vi "test TCX read (installed 71).vi"() -> ()   [LabVIEW 2011] (continued)
Position><AltitudeMeters>72.236</AltitudeMeters><DistanceMeters>5473.570</DistanceMeters><Cadence>72</Cadence><Extensions><TPX xmlns=\"http://www.garmin.com/xmlschemas/ActivityExtension/v2\"><Watts>158</Watts></TPX></Extensions></Trackpoint><Trackpoint><Time>2008-03-03T13:58:05Z</Time><Position><LatitudeDegrees>35.874487</LatitudeDegrees><LongitudeDegrees>-78.914089</LongitudeDegrees></Position><AltitudeMeters>72.236</AltitudeMeters><DistanceMeters>5483.258</DistanceMeters><Cadence>72</Cadence><Extensions><TPX xmlns=\"http://www.garmin.com/xmlschemas/ActivityExtension/v2\"><Watts>160</Watts></TPX></Extensions></Trackpoint><Trackpoint><Time>2008-03-03T13:58:06Z</Time><Position><LatitudeDegrees>35.874409</LatitudeDegrees><LongitudeDegrees>-78.914037</LongitudeDegrees></Position><AltitudeMeters>71.755</AltitudeMeters><DistanceMeters>5493.159</DistanceMeters><Cadence>73</Cadence><Extensions><TPX xmlns=\"http://www.garmin.com/xmlschemas/ActivityExtension/v2\"><Watts>157</Watts></TPX></Extensions></Trackpoint><Trackpoint><Time>2008-03-03T13:58:07Z</Time><Position><LatitudeDegrees>35.874330</LatitudeDegrees><LongitudeDegrees>-78.913985</LongitudeDegrees></Position><AltitudeMeters>72.236</AltitudeMeters><DistanceMeters>5503.068</DistanceMeters><Cadence>74</Cadence><Extensions><TPX xmlns=\"http://www.garmin.com/xmlschemas/ActivityExtension/v2\"><Watts>162</Watts></TPX></Extensions></Trackpoint><Trackpoint><Time>2008-03-03T13:58:08Z</Time><Position><LatitudeDegrees>35.874258</LatitudeDegrees><LongitudeDegrees>-78.913934</LongitudeDegrees></Position><AltitudeMeters>71.275</AltitudeMeters><DistanceMeters>5512.351</DistanceMeters><Cadence>75</Cadence><Extensions><TPX xmlns=\"http://www.garmin.com/xmlschemas/ActivityExtension/v2\"><Watts>156</Watts></TPX></Extensions></Trackpoint><Trackpoint><Time>2008-03-03T13:58:09Z</Time><Position><LatitudeDegrees>35.874185</LatitudeDegrees><LongitudeDegrees>-78.913883</LongitudeDegrees></Position><AltitudeMeters>71.755</AltitudeMeters><DistanceMeters>5521.553</DistanceMeters><Cadence>76</Cadence><Extensions><TPX xmlns=\"http://www.garmin.com/xmlschemas/ActivityExtension/v2\"><Watts>154</Watts></TPX></Extensions></Trackpoint><Trackpoint><Time>2008-03-03T13:58:10Z</Time><Position><LatitudeDegrees>35.874110</LatitudeDegrees><LongitudeDegrees>-78.913831</LongitudeDegrees></Position><AltitudeMeters>71.755</AltitudeMeters><DistanceMeters>5531.185</DistanceMeters><Cadence>76</Cadence><Extensions><TPX xmlns=\"http://www.garmin.com/xmlschemas/ActivityExtension/v2\"><Watts>152</Watts></TPX></Extensions></Trackpoint><Trackpoint><Time>2008-03-03T13:58:11Z</Time><Position><LatitudeDegrees>35.874038</LatitudeDegrees><LongitudeDegrees>-78.913777</LongitudeDegrees></Position><AltitudeMeters>71.755</AltitudeMeters><DistanceMeters>5540.583</DistanceMeters><Cadence>76</Cadence><Extensions><TPX xmlns=\"http://www.garmin.com/xmlschemas/ActivityExtension/v2\"><Watts>151</Watts></TPX></Extensions></Trackpoint><Trackpoint><Time>2008-03-03T13:58:12Z</Time><Position><LatitudeDegrees>35.873964</LatitudeDegrees><LongitudeDegrees>-78.913723</LongitudeDegrees></Position><AltitudeMeters>71.755</AltitudeMeters><DistanceMeters>5550.070</DistanceMeters><Cadence>76</Cadence><Extensions><TPX xmlns=\"http://www.garmin.com/xmlschemas/ActivityExtension/v2\"><Watts>149</Watts></TPX></Extensions></Trackpoint><Trackpoint><Time>2008-03-03T13:58:13Z</Time><Position><LatitudeDegrees>35.873889</LatitudeDegrees><LongitudeDegrees>-78.913669</LongitudeDegrees></Position><AltitudeMeters>71.275</AltitudeMeters><DistanceMeters>5559.694</DistanceMeters><Cadence>76</Cadence><Extensions><TPX xmlns=\"http://www.garmin.com/xmlschemas/ActivityExtension/v2\"><Watts>151</Watts></TPX></Extensions></Trackpoint><Trackpoint><Time>2008-03-03T13:58:14Z</Time><Position><LatitudeDegrees>35.873816</LatitudeDegrees><LongitudeDegrees>-78.913616</LongitudeDegrees></Position><AltitudeMeters>71.275</AltitudeMeters><DistanceMeters>5569.145</DistanceMeters><Cadence>75</Cadence><Extensions><TPX xmlns=\"http://www.garmin.com/xmlschemas/ActivityExtension/v2\"><Watts>155</Watts></TPX></Extensions></Trackpoint><Trackpoint><Time>2008-03-03T13:58:15Z</Time><Position><LatitudeDegrees>35.873721</LatitudeDegrees><LongitudeDegrees>-78.913558</LongitudeDegrees></Position><AltitudeMeters>71.275</AltitudeMeters><DistanceMeters>5580.802</DistanceMeters><Cadence>75</Cadence><Extensions><TPX xmlns=\"http://www.garmin.com/xmlschemas/ActivityExtension/v2\"><Watts>155</Watts></TPX></Extensions></Trackpoint><Trackpoint><Time>2008-03-03T13:58:16Z</Time><Position><LatitudeDegrees>35.873636</LatitudeDegrees><LongitudeDegrees>-78.913501</LongitudeDegrees></Position><AltitudeMeters>70.794</AltitudeMeters><DistanceMeters>5591.586</DistanceMeters><Cadence>75</Cadence><Extensions><TPX xmlns=\"http://www.garmin.com/xmlschemas/ActivityExtension/v2\"><Watts>169</Watts></TPX></Extensions></Trackpoint><Trackpoint><Time>2008-03-03T13:58:17Z</Time><Position><LatitudeDegrees>35.873565</LatitudeDegrees><LongitudeDegrees>-78.913457</LongitudeDegrees></Position><AltitudeMeters>70.313</AltitudeMeters><DistanceMeters>5600.361</DistanceMeters><Cadence>75</Cadence><Extensions><TPX xmlns=\"http://www.garmin.com/xmlschemas/ActivityExtension/v2\"><Watts>171</Watts></TPX></Extensions></Trackpoint><Trackpoint><Time>2008-03-03T13:58:18Z</Time><Position><LatitudeDegrees>35.873490</LatitudeDegrees><LongitudeDegrees>-78.913410</LongitudeDegrees></Position><AltitudeMeters>71.275</AltitudeMeters><DistanceMeters>5609.769</DistanceMeters><Cadence>74</Cadence><Extensions><TPX xmlns=\"http://www.garmin.com/xmlschemas/ActivityExtension/v2\"><Watts>171</Watts></TPX></Extensions></Trackpoint><Trackpoint><Time>2008-03-03T13:58:19Z</Time><Position><LatitudeDegrees>35.873403</LatitudeDegrees><LongitudeDegrees>-78.913362</LongitudeDegrees></Position><AltitudeMeters>71.275</AltitudeMeters><DistanceMeters>5620.357</DistanceMeters><Cadence>74</Cadence><Extensions><TPX xmlns=\"http://www.garmin.com/xmlschemas/ActivityExtension/v2\"><Watts>173</Watts></TPX></Extensions></Trackpoint><Trackpoint><Time>2008-03-03T13:58:20Z</Time><Position><LatitudeDegrees>35.873323</LatitudeDegrees><LongitudeDegrees>-78.913324</LongitudeDegrees></Position><AltitudeMeters>70.313</AltitudeMeters><DistanceMeters>5629.850</DistanceMeters><Cadence>74</Cadence><Extensions><TPX xmlns=\"http://www.garmin.com/xmlschemas/ActivityExtension/v2\"><Watts>173</Watts></TPX></Extensions></Trackpoint><Trackpoint><Time>2008-03-03T13:58:21Z</Time><Position><LatitudeDegrees>35.873230</LatitudeDegrees><LongitudeDegrees>-78.913281</LongitudeDegrees></Position><AltitudeMeters>70.794</AltitudeMeters><DistanceMeters>5640.867</DistanceMeters><Cadence>72</Cadence><Extensions><TPX xmlns=\"http://www.garmin.com/xmlschemas/ActivityExtension/v2\"><Watts>177</Watts></TPX></Extensions></Trackpoint><Trackpoint><Time>2008-03-03T13:58:22Z</Time><Position><LatitudeDegrees>35.873147</LatitudeDegrees><LongitudeDegrees>-78.913247</LongitudeDegrees></Position><AltitudeMeters>70.313</AltitudeMeters><DistanceMeters>5650.553</DistanceMeters><Cadence>72</Cadence><Extensions><TPX xmlns=\"http://www.garmin.com/xmlschemas/ActivityExtension/v2\"><Watts>177</Watts></TPX></Extensions></Trackpoint><Trackpoint><Time>2008-03-03T13:58:23Z</Time><Position><LatitudeDegrees>35.873063</LatitudeDegrees><LongitudeDegrees>-78.913217</LongitudeDegrees></Position><AltitudeMeters>70.313</AltitudeMeters><DistanceMeters>5660.292</DistanceMeters><Cadence>72</Cadence><Extensions><TPX xmlns=\"http://www.garmin.com/xmlschemas/ActivityExtension/v2\"><Watts>187</Watts></TPX></Extensions></Trackpoint><Trackpoint><Time>2008-03-03T13:58:24Z</Time><Position><LatitudeDegrees>35.872990</LatitudeDegrees><LongitudeDegrees>-78.913195</LongitudeDegrees></Position><AltitudeMeters>70.313</AltitudeMeters><DistanceMeters>5668.639</DistanceMeters><Cadence>71</Cadence><Extensions><TPX xmlns=\"http://www.garmin.com/xmlschemas/ActivityExtension/v2\"><Watts>195</Watts></TPX></Extensions></Trackpoint><Trackpoint><Time>2008-03-03T13:58:25Z</Time><Position><LatitudeDegrees>35.872909</LatitudeDegrees><LongitudeDegrees>-78.913177</LongitudeDegrees></Position><AltitudeMeters>69.833</AltitudeMeters><DistanceMeters>5677.786</DistanceMeters><Cadence>71</Cadence><Extensions><TPX xmlns=\"http://www.garmin.com/xmlschemas/ActivityExtension/v2\"><Watts>199</Watts></TPX></Extensions></Trackpoint><Trackpoint><Time>2008-03-03T13:58:26Z</Time><Position><LatitudeDegrees>35.872831</LatitudeDegrees><LongitudeDegrees>-78.913166</LongitudeDegrees></Position><AltitudeMeters>70.794</AltitudeMeters><DistanceMeters>5686.406</DistanceMeters><Cadence>70</Cadence><Extensions><TPX xmlns=\"http://www.garmin.com/xmlschemas/ActivityExtension/v2\"><Watts>233</Watts></TPX></Extensions></Trackpoint><Trackpoint><Time>2008-03-03T13:58:27Z</Time><Position><LatitudeDegrees>35.872755</LatitudeDegrees><LongitudeDegrees>-78.913161</LongitudeDegrees></Position><AltitudeMeters>70.794</AltitudeMeters><DistanceMeters>5694.925</DistanceMeters><Cadence>70</Cadence><Extensions><TPX xmlns=\"http://www.garmin.com/xmlschemas/ActivityExtension/v2\"><Watts>231</Watts></TPX></Extensions></Trackpoint><Trackpoint><Time>2008-03-03T13:58:28Z</Time><Position><LatitudeDegrees>35.872679</LatitudeDegrees><LongitudeDegrees>-78.913162</LongitudeDegrees></Position><AltitudeMeters>70.794</AltitudeMeters><DistanceMeters>5703.314</DistanceMeters><Cadence>68</Cadence><Extensions><TPX xmlns=\"http://www.garmin.com/xmlschemas/ActivityExtension/v2\"><Watts>242</Watts></TPX></Extensions></Trackpoint><Trackpoint><Time>2008-03-03T13:58:29Z</Time><Position><LatitudeDegrees>35.872603</LatitudeDegrees><LongitudeDegrees>-78.913168</LongitudeDegrees></Position><AltitudeMeters>71.275</AltitudeMeters><DistanceMeters>5711.774</DistanceMeters><Cadence>66</Cadence><Extensions><TPX xmlns=\"http://www.garmin.com/xmlschemas/ActivityExtension/v2\"><Watts>254</Watts></TPX></Extensions></Trackpoint><Trackpoint><Time>2008-03-03T13:58:30Z</Time><Position><LatitudeDegrees>35.872528</LatitudeDegrees><LongitudeDegrees>-78.913180</LongitudeDegrees></Position><AltitudeMeters>71.275</AltitudeMeters><DistanceMeters>5720.118</DistanceMeters><Cadence>66</Cadence><Extensions><TPX xmlns=\"http://www.garmin.com/xmlschemas/ActivityExtension/v2\"><Watts>274</Watts></TPX></Extensions></Trackpoint><Trackpoint><Time>2008-03-03T13:58:31Z</Time><Position><LatitudeDegrees>35.872454</LatitudeDegrees><LongitudeDegrees>-78.913197</LongitudeDegrees></Position><AltitudeMeters>71.275</AltitudeMeters><DistanceMeters>5728.521</DistanceMeters><Cadence>66</Cadence><Extensions><TPX xmlns=\"http://www.garmin.com/xmlschemas/ActivityExtension/v2\"><Watts>273</Watts></TPX></Extensions></Trackpoint><Trackpoint><Time>2008-03-03T13:58:32Z</Time><Position><LatitudeDegrees>35.872379</LatitudeDegrees><LongitudeDegrees>-78.913218</LongitudeDegrees></Position><AltitudeMeters>70.794</AltitudeMeters><DistanceMeters>5736.979</DistanceMeters><Cadence>65</Cadence><Extensions><TPX xmlns=\"http://www.garmin.com/xmlschemas/ActivityExtension/v2\"><Watts>271</Watts></TPX></Extensions></Trackpoint><Trackpoint><Time>2008-03-03T13:58:33Z</Time><Position><LatitudeDegrees>35.872306</LatitudeDegrees><LongitudeDegrees>-78.913239</LongitudeDegrees></Position><AltitudeMeters>70.794</AltitudeMeters><DistanceMeters>5745.323</DistanceMeters><Cadence>66</Cadence><Extensions><TPX xmlns=\"http://www.garmin.com/xmlschemas/ActivityExtension/v2\"><Watts>258</Watts></TPX></Extensions></Trackpoint><Trackpoint><Time>2008-03-03T13:58:34Z</Time><Position><LatitudeDegrees>35.872233</LatitudeDegrees><LongitudeDegrees>-78.913259</LongitudeDegrees></Position><AltitudeMeters>70.794</AltitudeMeters><DistanceMeters>5753.588</DistanceMeters><Cadence>65</Cadence><Extensions><TPX xmlns=\"http://www.garmin.com/xmlschemas/ActivityExtension/v2\"><Watts>215</Watts></TPX></Extensions></Trackpoint><Trackpoint><Time>2008-03-03T13:58:35Z</Time><Position><LatitudeDegrees>35.872160</LatitudeDegrees><LongitudeDegrees>-78.913281</LongitudeDegrees></Position><AltitudeMeters>70.794</AltitudeMeters><DistanceMeters>5761.984</DistanceMeters><Cadence>67</Cadence><Extensions><TPX xmlns=\"http://www.garmin.com/xmlschemas/ActivityExtension/v2\"><Watts>260</Watts></TPX></Extensions></Trackpoint><Trackpoint><Time>2008-03-03T13:58:36Z</Time><Position><LatitudeDegrees>35.872087</LatitudeDegrees><LongitudeDegrees>-78.913302</LongitudeDegrees></Position><AltitudeMeters>71.755</AltitudeMeters><DistanceMeters>5770.306</DistanceMeters><Cadence>66</Cadence><Extensions><TPX xmlns=\"http://www.garmin.com/xmlschemas/ActivityExtension/v2\"><Watts>213</Watts></TPX></Extensions></Trackpoint><Trackpoint><Time>2008-03-03T13:58:37Z</Time><Position><LatitudeDegrees>35.872009</LatitudeDegrees><LongitudeDegrees>-78.913321</LongitudeDegrees></Position><AltitudeMeters>71.275</AltitudeMeters><DistanceMeters>5779.111</DistanceMeters><Cadence>66</Cadence><Extensions><TPX xmlns=\"http://www.garmin.com/xmlschemas/ActivityExtension/v2\"><Watts>217</Watts></TPX></Extensions></Trackpoint><Trackpoint><Time>2008-03-03T13:58:38Z</Time><Position><LatitudeDegrees>35.871937</LatitudeDegrees><LongitudeDegrees>-78.913345</LongitudeDegrees></Position><AltitudeMeters>71.275</AltitudeMeters><DistanceMeters>5787.370</DistanceMeters><Cadence>65</Cadence><Extensions><TPX xmlns=\"http://www.garmin.com/xmlschemas/ActivityExtension/v2\"><Watts>193</Watts></TPX></Extensions></Trackpoint><Trackpoint><Time>2008-03-03T13:58:39Z</Time><Position><LatitudeDegrees>35.871870</LatitudeDegrees><LongitudeDegrees>-78.913372</LongitudeDegrees></Position><AltitudeMeters>71.275</AltitudeMeters><DistanceMeters>5795.163</DistanceMeters><Cadence>65</Cadence><Extensions><TPX xmlns=\"http://www.garmin.com/xmlschemas/ActivityExtension/v2\"><Watts>194</Watts></TPX></Extensions></Trackpoint><Trackpoint><Time>2008-03-03T13:58:40Z</Time><Position><LatitudeDegrees>35.871808</LatitudeDegrees><LongitudeDegrees>-78.913401</LongitudeDegrees></Position><AltitudeMeters>71.755</AltitudeMeters><DistanceMeters>5802.564</DistanceMeters><Cadence>65</Cadence><Extensions><TPX xmlns=\"http://www.garmin.com/xmlschemas/ActivityExtension/v2\"><Watts>192</Watts></TPX></Extensions></Trackpoint><Trackpoint><Time>2008-03-03T13:58:41Z</Time><Position><LatitudeDegrees>35.871744</LatitudeDegrees><LongitudeDegrees>-78.913433</LongitudeDegrees></Position><AltitudeMeters>71.275</AltitudeMeters><DistanceMeters>5810.239</DistanceMeters><Cadence>63</Cadence><Extensions><TPX xmlns=\"http://www.garmin.com/xmlschemas/ActivityExtension/v2\"><Watts>207</Watts></TPX></Extensions></Trackpoint><Trackpoint><Time>2008-03-03T13:58:42Z</Time><Position><LatitudeDegrees>35.871679</LatitudeDegrees><LongitudeDegrees>-78.913464</LongitudeDegrees></Position><AltitudeMeters>71.755</AltitudeMeters><DistanceMeters>5817.914</DistanceMeters><Cadence>61</Cadence><Extensions><TPX xmlns=\"http://www.garmin.com/xmlschemas/ActivityExtension/v2\"><Watts>197</Watts></TPX></Extensions></Trackpoint><Trackpoint><Time>2008-03-03T13:58:43Z</Time><Position><LatitudeDegrees>35.871618</LatitudeDegrees><LongitudeDegrees>-78.913494</LongitudeDegrees></Position><AltitudeMeters>72.236</AltitudeMeters><DistanceMeters>5825.149</DistanceMeters><Cadence>62</Cadence><Extensions><TPX xmlns=\"http://www.garmin.com/xmlschemas/ActivityExtension/v2\"><Watts>201</Watts></TPX></Extensions></Trackpoint><Trackpoint><Time>2008-03-03T13:58:44Z</Time><Position><LatitudeDegrees>35.871558</LatitudeDegrees><LongitudeDegrees>-78.913527</LongitudeDegrees></Position><AltitudeMeters>72.236</AltitudeMeters><DistanceMeters>5832.490</DistanceMeters><Cadence>69</Cadence><Extensions><TPX xmlns=\"http://www.garmin.com/xmlschemas/ActivityExtension/v2\"><Watts>203</Watts></TPX></Extensions></Trackpoint><Trackpoint><Time>2008-03-03T13:58:45Z</Time><Position><LatitudeDegrees>35.871498</LatitudeDegrees><LongitudeDegrees>-78.913560</LongitudeDegrees></Position><AltitudeMeters>72.717</AltitudeMeters><DistanceMeters>5839.716</DistanceMeters><Cadence>68</Cadence><Extensions><TPX xmlns=\"http://www.garmin.com/xmlschemas/ActivityExtension/v2\"><Watts>328</Watts></TPX></Extensions></Trackpoint><Trackpoint><Time>2008-03-03T13:58:46Z</Time><Position><LatitudeDegrees>35.871438</LatitudeDegrees><LongitudeDegrees>-78.913592</LongitudeDegrees></Position><AltitudeMeters>72.717</AltitudeMeters><DistanceMeters>5847.000</DistanceMeters><Cadence>68</Cadence><Extensions><TPX xmlns=\"http://www.garmin.com/xmlschemas/ActivityExtension/v2\"><Watts>327</Watts></TPX></Extensions></Trackpoint><Trackpoint><Time>2008-03-03T13:58:47Z</Time><Position><LatitudeDegrees>35.871382</LatitudeDegrees><LongitudeDegrees>-78.913626</LongitudeDegrees></Position><AltitudeMeters>73.198</AltitudeMeters><DistanceMeters>5853.856</DistanceMeters><Cadence>69</Cadence><Extensions><TPX xmlns=\"http://www.garmin.com/xmlschemas/ActivityExtension/v2\"><Watts>441</Watts></TPX></Extensions></Trackpoint><Trackpoint><Time>2008-03-03T13:58:48Z</Time><Position><LatitudeDegrees>35.871325</LatitudeDegrees><LongitudeDegrees>-78.913660</LongitudeDegrees></Position><AltitudeMeters>73.678</AltitudeMeters><DistanceMeters>5860.916</DistanceMeters><Cadence>69</Cadence><Extensions><TPX xmlns=\"http://www.garmin.com/xmlschemas/ActivityExtension/v2\"><Watts>452</Watts></TPX></Extensions></Trackpoint><Trackpoint><Time>2008-03-03T13:58:49Z</Time><Position><LatitudeDegrees>35.871269</LatitudeDegrees><LongitudeDegrees>-78.913693</LongitudeDegrees></Position><AltitudeMeters>74.159</AltitudeMeters><DistanceMeters>5867.837</DistanceMeters><Cadence>68</Cadence><Extensions><TPX xmlns=\"http://www.garmin.com/xmlschemas/ActivityExtension/v2\"><Watts>455</Watts></TPX></Extensions></Trackpoint><Trackpoint><Time>2008-03-03T13:58:50Z</Time><Position><LatitudeDegrees>35.871212</LatitudeDegrees><LongitudeDegrees>-78.913724</LongitudeDegrees></Position><AltitudeMeters>74.159</AltitudeMeters><DistanceMeters>5874.745</DistanceMeters><Cadence>67</Cadence><Extensions><TPX xmlns=\"http://www.garmin.com/xmlschemas/ActivityExtension/v2\"><Watts>419</Watts></TPX></Extensions></Trackpoint><Trackpoint><Time>2008-03-03T13:58:51Z</Time><Position><LatitudeDegrees>35.871157</LatitudeDegrees><LongitudeDegrees>-78.913754</LongitudeDegrees></Position><AltitudeMeters>74.640</AltitudeMeters><DistanceMeters>5881.423</DistanceMeters><Cadence>65</Cadence><Extensions><TPX xmlns=\"http://www.garmin.com/xmlschemas/ActivityExtension/v2\"><Watts>392</Watts></TPX></Extensions></Trackpoint><Trackpoint><Time>2008-03-03T13:58:52Z</Time><Position><LatitudeDegrees>35.871099</LatitudeDegrees><LongitudeDegrees>-78.913784</LongitudeDegrees></Position><AltitudeMeters>75.120</AltitudeMeters><DistanceMeters>5888.344</DistanceMeters><Cadence>65</Cadence><Extensions><TPX xmlns=\"http://www.garmin.com/xmlschemas/ActivityExtension/v2\"><Watts>388</Watts></TPX></Extensions></Trackpoint><Trackpoint><Time>2008-03-03T13:58:53Z</Time><Position><LatitudeDegrees>35.871043</LatitudeDegrees><LongitudeDegrees>-78.913814</LongitudeDegrees></Position><AltitudeMeters>75.120</AltitudeMeters><DistanceMeters>5895.120</DistanceMeters><Cadence>64</Cadence><Extensions><TPX xmlns=\"http://www.garmin.com/xmlschemas/ActivityExtension/v2\"><Watts>393</Watts></TPX></Extensions></Trackpoint><Trackpoint><Time>2008-03-03T13:58:54Z</Time><Position><LatitudeDegrees>35.870990</LatitudeDegrees><LongitudeDegrees>-78.913846</LongitudeDegrees></Position><AltitudeMeters>75.601</AltitudeMeters><DistanceMeters>5901.719</DistanceMeters><Cadence>65</Cadence><Extensions><TPX xmlns=\"http://www.garmin.com/xmlschemas/ActivityExtension/v2\"><Watts>408</Watts></TPX></Extensions></Trackpoint><Trackpoint><Time>2008-03-03T13:58:55Z</Time><Position><LatitudeDegrees>35.870935</LatitudeDegrees><LongitudeDegrees>-78.913877</LongitudeDegrees></Position><AltitudeMeters>76.081</AltitudeMeters><DistanceMeters>5908.360</DistanceMeters><Cadence>64</Cadence><Extensions><TPX xmlns=\"http://www.garmin.com/xmlschemas/ActivityExtension/v2\"><Watts>404</Watts></TPX></Extensions></Trackpoint><Trackpoint><Time>2008-03-03T13:58:56Z</Time><Position><LatitudeDegrees>35.870883</LatitudeDegrees><LongitudeDegrees>-78.913908</LongitudeDegrees></Position><AltitudeMeters>76.081</AltitudeMeters><DistanceMeters>5914.815</DistanceMeters><Cadence>63</Cadence><Extensions><TPX xmlns=\"http://www.garmin.com/xmlschemas/ActivityExtension/v2\"><Watts>380</Watts></TPX></Extensions></Trackpoint><Trackpoint><Time>2008-03-03T13:58:57Z</Time><Position><LatitudeDegrees>35.870832</LatitudeDegrees><LongitudeDegrees>-78.913940</LongitudeDegrees></Position><AltitudeMeters>76.562</AltitudeMeters><DistanceMeters>5921.137</DistanceMeters><Cadence>63</Cadence><Extensions><TPX xmlns=\"http://www.garmin.com/xmlschemas/ActivityExtension/v2\"><Watts>385</Watts></TPX></Extensions></Trackpoint><Trackpoint><Time>2008-03-03T13:58:58Z</Time><Position><LatitudeDegrees>35.870775</LatitudeDegrees><LongitudeDegrees>-78.913971</LongitudeDegrees></Position><AltitudeMeters>77.043</AltitudeMeters><DistanceMeters>5928.036</DistanceMeters><Cadence>63</Cadence><Extensions><TPX xmlns=\"http://www.garmin.com/xmlschemas/ActivityExtension/v2\"><Watts>374</Watts></TPX></Extensions></Trackpoint><Trackpoint><Time>2008-03-03T13:58:59Z</Time><Position><LatitudeDegrees>35.870720</LatitudeDegrees><LongitudeDegrees>-78.914001</LongitudeDegrees></Position><AltitudeMeters>77.043</AltitudeMeters><DistanceMeters>5934.812</DistanceMeters><Cadence>63</Cadence><Extensions><TPX xmlns=\"http://www.garmin.com/xmlschemas/ActivityExtension/v2\"><Watts>378</Watts></TPX></Extensions></Trackpoint><Trackpoint><Time>2008-03-03T13:59:00Z</Time><Position><LatitudeDegrees>35.870655</LatitudeDegrees><LongitudeDegrees>-78.914027</LongitudeDegrees></Position><AltitudeMeters>77.043</AltitudeMeters><DistanceMeters>5942.442</DistanceMeters><Cadence>63</Cadence><Extensions><TPX xmlns=\"http://www.garmin.com/xmlschemas/ActivityExtension/v2\"><Watts>391</Watts></TPX></Extensions></Trackpoint><Trackpoint><Time>2008-03-03T13:59:01Z</Time><Position><LatitudeDegrees>35.870596</LatitudeDegrees><LongitudeDegrees>-78.914056</LongitudeDegrees></Position><AltitudeMeters>77.523</AltitudeMeters><DistanceMeters>5949.411</DistanceMeters><Cadence>64</Cadence><Extensions><TPX xmlns=\"http://www.garmin.com/xmlschemas/ActivityExtension/v2\"><Watts>391</Watts></TPX></Extensions></Trackpoint><Trackpoint><Time>2008-03-03T13:59:02Z</Time><Position><LatitudeDegrees>35.870541</LatitudeDegrees><LongitudeDegrees>-78.914088</LongitudeDegrees></Position><AltitudeMeters>78.004</AltitudeMeters><DistanceMeters>5956.139</DistanceMeters><Cadence>64</Cadence><Extensions><TPX xmlns=\"http://www.garmin.com/xmlschemas/ActivityExtension/v2\"><Watts>392</Watts></TPX></Extensions></Trackpoint><Trackpoint><Time>2008-03-03T13:59:03Z</Time><Position><LatitudeDegrees>35.870486</LatitudeDegrees><LongitudeDegrees>-78.914120</LongitudeDegrees></Position><AltitudeMeters>78.004</AltitudeMeters><DistanceMeters>5962.949</DistanceMeters><Cadence>65</Cadence><Extensions><TPX xmlns=\"http://www.garmin.com/xmlschemas/ActivityExtension/v2\"><Watts>371</Watts></TPX></Extensions></Trackpoint><Trackpoint><Time>2008-03-03T13:59:04Z</Time><Position><LatitudeDegrees>35.870427</LatitudeDegrees><LongitudeDegrees>-78.914151</LongitudeDegrees></Position><AltitudeMeters>78.485</AltitudeMeters><DistanceMeters>5969.976</DistanceMeters><Cadence>65</Cadence><Extensions><TPX xmlns=\"http://www.garmin.com/xmlschemas/ActivityExtension/v2\"><Watts>368</Watts></TPX></Extensions></Trackpoint><Trackpoint><Time>2008-03-03T13:59:05Z</Time><Position><LatitudeDegrees>35.870366</LatitudeDegrees><LongitudeDegrees>-78.914180</LongitudeDegrees></Position><AltitudeMeters>78.485</AltitudeMeters><DistanceMeters>5977.312</DistanceMeters><Cadence>66</Cadence><Extensions><TPX xmlns=\"http://www.garmin.com/xmlschemas/ActivityExtension/v2\"><Watts>361</Watts></TPX></Extensions></Trackpoint><Trackpoint><Time>2008-03-03T13:59:06Z</Time><Position><LatitudeDegrees>35.870309</LatitudeDegrees><LongitudeDegrees>-78.914212</LongitudeDegrees></Position><AltitudeMeters>78.965</AltitudeMeters><DistanceMeters>5984.270</DistanceMeters><Cadence>66</Cadence><Extensions><TPX xmlns=\"http://www.garmin.com/xmlschemas/ActivityExtension/v2\"><Watts>358</Watts></TPX></Extensions></Trackpoint><Trackpoint><Time>2008-03-03T13:59:07Z</Time><Position><LatitudeDegrees>35.870252</LatitudeDegrees><LongitudeDegrees>-78.914244</LongitudeDegrees></Position><AltitudeMeters>79.446</AltitudeMeters><DistanceMeters>5991.213</DistanceMeters><Cadence>64</Cadence><Extensions><TPX xmlns=\"http://www.garmin.com/xmlschemas/ActivityExtension/v2\"><Watts>327</Watts></TPX></Extensions></Trackpoint><Trackpoint><Time>2008-03-03T13:59:08Z</Time><Position><LatitudeDegrees>35.870192</LatitudeDegrees><LongitudeDegrees>-78.914274</LongitudeDegrees></Position><AltitudeMeters>79.446</AltitudeMeters><DistanceMeters>5998.372</DistanceMeters><Cadence>64</Cadence><Extensions><TPX xmlns=\"http://www.garmin.com/xmlschemas/ActivityExtension/v2\"><Watts>318</Watts></TPX></Extensions></Trackpoint><Trackpoint><Time>2008-03-03T13:59:09Z</Time><Position><LatitudeDegrees>35.870131</LatitudeDegrees><LongitudeDegrees>-78.914304</LongitudeDegrees></Position><AltitudeMeters>79.446</AltitudeMeters><DistanceMeters>6005.639</DistanceMeters><Cadence>64</Cadence><Extensions><TPX xmlns=\"http://www.garmin.com/xmlschemas/ActivityExtension/v2\"><Watts>317</Watts></TPX></Extensions></Trackpoint><Trackpoint><Time>2008-03-03T13:59:10Z</Time><Position><LatitudeDegrees>35.870070</LatitudeDegrees><LongitudeDegrees>-78.914334</LongitudeDegrees></Position><AltitudeMeters>79.927</AltitudeMeters><DistanceMeters>6012.941</DistanceMeters><Cadence>65</Cadence><Extensions><TPX xmlns=\"http://www.garmin.com/xmlschemas/ActivityExtension/v2\"><Watts>317</Watts></TPX></Extensions></Trackpoint><Trackpoint><Time>2008-03-03T13:59:11Z</Time><Position><LatitudeDegrees>35.870010</LatitudeDegrees><LongitudeDegrees>-78.914365</LongitudeDegrees></Position><AltitudeMeters>79.927</AltitudeMeters><DistanceMeters>6020.168</DistanceMeters><Cadence>65</Cadence><Extensions><TPX xmlns=\"http://www.garmin.com/xmlschemas/ActivityExtension/v2\"><Watts>319</Watts></TPX></Extensions></Trackpoint><Trackpoint><Time>2008-03-03T13:59:12Z</Time><Position><LatitudeDegrees>35.869949</LatitudeDegrees><LongitudeDegrees>-78.914395</LongitudeDegrees></Position><AltitudeMeters>79.927</AltitudeMeters><DistanceMeters>6027.465</DistanceMeters><Cadence>65</Cadence><Extensions><TPX xmlns=\"http://www.garmin.com/xmlschemas/ActivityExtension/v2\"><Watts>294</Watts></TPX></Extensions></Trackpoint><Trackpoint><Time>2008-03-03T13:59:13Z</Time><Position><LatitudeDegrees>35.869890</LatitudeDegrees><LongitudeDegrees>-78.914426</LongitudeDegrees></Position><AltitudeMeters>79.927</AltitudeMeters><DistanceMeters>6034.622</DistanceMeters><Cadence>65</Cadence><Extensions><TPX xmlns=\"http://www.garmin.com/xmlschemas/ActivityExtension/v2\"><Watts>270</Watts></TPX></Extensions></Trackpoint><Trackpoint><Time>2008-03-03T13:59:14Z</Time><Position><LatitudeDegrees>35.869830</LatitudeDegrees><LongitudeDegrees>-78.914457</LongitudeDegrees></Position><AltitudeMeters>80.407</AltitudeMeters><DistanceMeters>6041.830</DistanceMeters><Cadence>65</Cadence><Extensions><TPX xmlns=\"http://www.garmin.com/xmlschemas/ActivityExtension/v2\"><Watts>268</Watts></TPX></Extensions></Trackpoint><Trackpoint><Time>2008-03-03T13:59:15Z</Time><Position><LatitudeDegrees>35.869769</LatitudeDegrees><LongitudeDegrees>-78.914487</LongitudeDegrees></Position><AltitudeMeters>80.407</AltitudeMeters><DistanceMeters>6049.062</DistanceMeters><Cadence>65</Cadence><Extensions><TPX xmlns=\"http://www.garmin.com/xmlschemas/ActivityExtension/v2\"><Watts>233</Watts></TPX></Extensions></Trackpoint><Trackpoint><Time>2008-03-03T13:59:16Z</Time><Position><LatitudeDegrees>35.869708</LatitudeDegrees><LongitudeDegrees>-78.914516</LongitudeDegrees></Position><AltitudeMeters>80.407</AltitudeMeters><DistanceMeters>6056.318</DistanceMeters><Cadence>65</Cadence><Extensions><TPX xmlns=\"http://www.garmin.com/xmlschemas/ActivityExtension/v2\"><Watts>233</Watts></TPX></Extensions></Trackpoint><Trackpoint><Time>2008-03-03T13:59:17Z</Time><Position><LatitudeDegrees>35.869647</LatitudeDegrees><LongitudeDegrees>-78.914545</LongitudeDegrees></Position><AltitudeMeters>80.888</AltitudeMeters><DistanceMeters>6063.643</DistanceMeters><Cadence>66</Cadence><Extensions><TPX xmlns=\"http://www.garmin.com/xmlschemas/ActivityExtension/v2\"><Watts>244</Watts></TPX></Extensions></Trackpoint><Trackpoint><Time>2008-03-03T13:59:18Z</Time><Position><LatitudeDegrees>35.869589</LatitudeDegrees><LongitudeDegrees>-78.914573</LongitudeDegrees></Position><AltitudeMeters>80.888</AltitudeMeters><DistanceMeters>6070.584</DistanceMeters><Cadence>66</Cadence><Extensions><TPX xmlns=\"http://www.garmin.com/xmlschemas/ActivityExtension/v2\"><Watts>219</Watts></TPX></Extensions></Trackpoint><Trackpoint><Time>2008-03-03T13:59:19Z</Time><Position><LatitudeDegrees>35.869530</LatitudeDegrees><LongitudeDegrees>-78.914600</LongitudeDegrees></Position><AltitudeMeters>80.888</AltitudeMeters><DistanceMeters>6077.537</DistanceMeters><Cadence>66</Cadence><Extensions><TPX xmlns=\"http://www.garmin.com/xmlschemas/ActivityExtension/v2\"><Watts>202</Watts></TPX></Extensions></Trackpoint><Trackpoint><Time>2008-03-03T13:59:20Z</Time><Position><LatitudeDegrees>35.869468</LatitudeDegrees><LongitudeDegrees>-78.914624</LongitudeDegrees></Position><AltitudeMeters>80.888</AltitudeMeters><DistanceMeters>6084.710</DistanceMeters><Cadence>66</Cadence><Extensions><TPX xmlns=\"http://www.garmin.com/xmlschemas/ActivityExtension/v2\"><Watts>195</Watts></TPX></Extensions></Trackpoint><Trackpoint><Time>2008-03-03T13:59:21Z</Time><Position><LatitudeDegrees>35.869406</LatitudeDegrees><LongitudeDegrees>-78.914646</LongitudeDegrees></Position><AltitudeMeters>80.888</AltitudeMeters><DistanceMeters>6091.856</DistanceMeters><Cadence>66</Cadence><Extensions><TPX xmlns=\"http://www.garmin.com/xmlschemas/ActivityExtension/v2\"><Watts>196</Watts></TPX></Extensions></Trackpoint><Trackpoint><Time>2008-03-03T13:59:22Z</Time><Position><LatitudeDegrees>35.869344</LatitudeDegrees><LongitudeDegrees>-78.914668</LongitudeDegrees></Position><AltitudeMeters>80.888</AltitudeMeters><DistanceMeters>6099.025</DistanceMeters><Cadence>66</Cadence><Extensions><TPX xmlns=\"http://www.garmin.com/xmlschemas/ActivityExtension/v2\"><Watts>177</Watts></TPX></Extensions></Trackpoint><Trackpoint><Time>2008-03-03T13:59:23Z</Time><Position><LatitudeDegrees>35.869282</LatitudeDegrees><LongitudeDegrees>-78.914689</LongitudeDegrees></Position><AltitudeMeters>81.369</AltitudeMeters><DistanceMeters>6106.212</DistanceMeters><Cadence>66</Cadence><Extensions><TPX xmlns=\"http://www.garmin.com/xmlschemas/ActivityExtension/v2\"><Watts>171</Watts></TPX></Extensions></Trackpoint><Trackpoint><Time>2008-03-03T13:59:24Z</Time><Position><LatitudeDegrees>35.869221</LatitudeDegrees><LongitudeDegrees>-78.914707</LongitudeDegrees></Position><AltitudeMeters>81.369</AltitudeMeters><DistanceMeters>6113.151</DistanceMeters><Cadence>66</Cadence><Extensions><TPX xmlns=\"http://www.garmin.com/xmlschemas/ActivityExtension/v2\"><Watts>176</Watts></TPX></Extensions></Trackpoint><Trackpoint><Time>2008-03-03T13:59:25Z</Time><Position><LatitudeDegrees>35.869155</LatitudeDegrees><LongitudeDegrees>-78.914722</LongitudeDegrees></Position><AltitudeMeters>81.369</AltitudeMeters><DistanceMeters>6120.588</DistanceMeters><Cadence>67</Cadence><Extensions><TPX xmlns=\"http://www.garmin.com/xmlschemas/ActivityExtension/v2\"><Watts>176</Watts></TPX></Extensions></Trackpoint><Trackpoint><Time>2008-03-03T13:59:26Z</Time><Position><LatitudeDegrees>35.869090</LatitudeDegrees><LongitudeDegrees>-78.914736</LongitudeDegrees></Position><AltitudeMeters>80.888</AltitudeMeters><DistanceMeters>6127.882</DistanceMeters><Cadence>67</Cadence><Extensions><TPX xmlns=\"http://www.garmin.com/xmlschemas/ActivityExtension/v2\"><Watts>159</Watts></TPX></Extensions></Trackpoint><Trackpoint><Time>2008-03-03T13:59:27Z</Time><Position><LatitudeDegrees>35.869025</LatitudeDegrees><LongitudeDegrees>-78.914746</LongitudeDegrees></Position><AltitudeMeters>80.888</AltitudeMeters><DistanceMeters>6135.227</DistanceMeters><Cadence>67</Cadence><Extensions><TPX xmlns=\"http://www.garmin.com/xmlschemas/ActivityExtension/v2\"><Watts>143</Watts></TPX></Extensions></Trackpoint><Trackpoint><Time>2008-03-03T13:59:28Z</Time><Position><LatitudeDegrees>35.868959</LatitudeDegrees><LongitudeDegrees>-78.914755</LongitudeDegrees></Position><AltitudeMeters>80.888</AltitudeMeters><DistanceMeters>6142.568</DistanceMeters><Cadence>68</Cadence><Extensions><TPX xmlns=\"http://www.garmin.com/xmlschemas/ActivityExtension/v2\"><Watts>142</Watts></TPX></Extensions></Trackpoint><Trackpoint><Time>2008-03-03T13:59:29Z</Time><Position><LatitudeDegrees>35.868895</LatitudeDegrees><LongitudeDegrees>-78.914761</LongitudeDegrees></Position><AltitudeMeters>80.888</AltitudeMeters><DistanceMeters>6149.737</DistanceMeters><Cadence>68</Cadence><Extensions><TPX xmlns=\"http://www.garmin.com/xmlschemas/ActivityExtension/v2\"><Watts>144</Watts></TPX></Extensions></Trackpoint><Trackpoint><Time>2008-03-03T13:59:30Z</Time><Position><LatitudeDegrees>35.868828</LatitudeDegrees><LongitudeDegrees>-78.914768</LongitudeDegrees></Position><AltitudeMeters>80.888</AltitudeMeters><DistanceMeters>6157.170</DistanceMeters><Cadence>69</Cadence><Extensions><TPX xmlns=\"http://www.garmin.com/xmlschemas/ActivityExtension/v2\"><Watts>145</Watts></TPX></Extensions></Trackpoint><Trackpoint><Time>2008-03-03T13:59:31Z</Time><Position><LatitudeDegrees>35.868761</LatitudeDegrees><LongitudeDegrees>-78.914773</LongitudeDegrees></Position><AltitudeMeters>80.888</AltitudeMeters><DistanceMeters>6164.539</DistanceMeters><Cadence>69</Cadence><Extensions><TPX xmlns=\"http://www.garmin.com/xmlschemas/ActivityExtension/v2\"><Watts>144</Watts></TPX></Extensions></Trackpoint><Trackpoint><Time>2008-03-03T13:59:32Z</Time><Position><LatitudeDegrees>35.868695</LatitudeDegrees><LongitudeDegrees>-78.914777</LongitudeDegrees></Position><AltitudeMeters>80.888</AltitudeMeters><DistanceMeters>6171.962</DistanceMeters><Cadence>69</Cadence><Extensions><TPX xmlns=\"http://www.garmin.com/xmlschemas/ActivityExtension/v2\"><Watts>146</Watts></TPX></Extensions></Trackpoint><Trackpoint><Time>2008-03-03T13:59:33Z</Time><Position><LatitudeDegrees>35.868627</LatitudeDegrees><LongitudeDegrees>-78.914779</LongitudeDegrees></Position><AltitudeMeters>81.369</AltitudeMeters><DistanceMeters>6179.457</DistanceMeters><Cadence>69</Cadence><Extensions><TPX xmlns=\"http://www.garmin.com/xmlschemas/ActivityExtension/v2\"><Watts>146</Watts></TPX></Extensions></Trackpoint><Trackpoint><Time>2008-03-03T13:59:34Z</Time><Position><LatitudeDegrees>35.868560</LatitudeDegrees><LongitudeDegrees>-78.914779</LongitudeDegrees></Position><AltitudeMeters>81.369</AltitudeMeters><DistanceMeters>6186.896</DistanceMeters><Cadence>69</Cadence><Extensions><TPX xmlns=\"http://www.garmin.com/xmlschemas/ActivityExtension/v2\"><Watts>146</Watts></TPX></Extensions></Trackpoint><Trackpoint><Time>2008-03-03T13:59:35Z</Time><Position><LatitudeDegrees>35.868492</LatitudeDegrees><LongitudeDegrees>-78.914779</LongitudeDegrees></Position><AltitudeMeters>81.369</AltitudeMeters><DistanceMeters>6194.394</DistanceMeters><Cadence>69</Cadence><Extensions><TPX xmlns=\"http://www.garmin.com/xmlschemas/ActivityExtension/v2\"><Watts>139</Watts></TPX></Extensions></Trackpoint><Trackpoint><Time>2008-03-03T13:59:36Z</Time><Position><LatitudeDegrees>35.868426</LatitudeDegrees><LongitudeDegrees>-78.914782</LongitudeDegrees></Position><AltitudeMeters>81.369</AltitudeMeters><DistanceMeters>6201.778</DistanceMeters><Cadence>69</Cadence><Extensions><TPX xmlns=\"http://www.garmin.com/xmlschemas/ActivityExtension/v2\"><Watts>138</Watts></TPX></Extensions></Trackpoint><Trackpoint><Time>2008-03-03T13:59:37Z</Time><Position><LatitudeDegrees>35.868358</LatitudeDegrees><LongitudeDegrees>-78.914783</LongitudeDegrees></Position><AltitudeMeters>81.369</AltitudeMeters><DistanceMeters>6209.298</DistanceMeters><Cadence>68</Cadence><Extensions><TPX xmlns=\"http://www.garmin.com/xmlschemas/ActivityExtension/v2\"><Watts>142</Watts></TPX></Extensions></Trackpoint><Trackpoint><Time>2008-03-03T13:59:38Z</Time><Position><LatitudeDegrees>35.868290</LatitudeDegrees><LongitudeDegrees>-78.914783</LongitudeDegrees></Position><AltitudeMeters>81.369</AltitudeMeters><DistanceMeters>6216.898</DistanceMeters><Cadence>68</Cadence><Extensions><TPX xmlns=\"http://www.garmin.com/xmlschemas/ActivityExtension/v2\"><Watts>150</Watts></TPX></Extensions></Trackpoint><Trackpoint><Time>2008-03-03T13:59:39Z</Time><Position><LatitudeDegrees>35.868223</LatitudeDegrees><LongitudeDegrees>-78.914783</LongitudeDegrees></Position><AltitudeMeters>81.849</AltitudeMeters><DistanceMeters>6224.316</DistanceMeters><Cadence>68</Cadence><Extensions><TPX xmlns=\"http://www.garmin.com/xmlschemas/ActivityExtension/v2\"><Watts>159</Watts></TPX></Extensions></Trackpoint><Trackpoint><Time>2008-03-03T13:59:40Z</Time><Position><LatitudeDegrees>35.868157</LatitudeDegrees><LongitudeDegrees>-78.914784</LongitudeDegrees></Position><AltitudeMeters>81.849</AltitudeMeters><DistanceMeters>6231.565</DistanceMeters><Cadence>68</Cadence><Extensions><TPX xmlns=\"http://www.garmin.com/xmlschemas/ActivityExtension/v2\"><Watts>159</Watts></TPX></Extensions></Trackpoint><Trackpoint><Time>2008-03-03T13:59:41Z</Time><Position><LatitudeDegrees>35.868093</LatitudeDegrees><LongitudeDegrees>-78.914785</LongitudeDegrees></Position><AltitudeMeters>81.849</AltitudeMeters><DistanceMeters>6238.785</DistanceMeters><Cadence>67</Cadence><Extensions><TPX xmlns=\"http://www.garmin.com/xmlschemas/ActivityExtension/v2\"><Watts>168</Watts></TPX></Extensions></Trackpoint><Trackpoint><Time>2008-03-03T13:59:42Z</Time><Position><LatitudeDegrees>35.868028</LatitudeDegrees><LongitudeDegrees>-78.914787</LongitudeDegrees></Position><AltitudeMeters>81.849</AltitudeMeters><DistanceMeters>6245.958</DistanceMeters><Cadence>67</Cadence><Extensions><TPX xmlns=\"http://www.garmin.com/xmlschemas/ActivityExtension/v2\"><Watts>158</Watts></TPX></Extensions></Trackpoint><Trackpoint><Time>2008-03-03T13:59:43Z</Time><Position><LatitudeDegrees>35.867963</LatitudeDegrees><LongitudeDegrees>-78.914789</LongitudeDegrees></Position><AltitudeMeters>81.849</AltitudeMeters><DistanceMeters>6253.119</DistanceMeters><Cadence>67</Cadence><Extensions><TPX xmlns=\"http://www.garmin.com/xmlschemas/ActivityExtension/v2\"><Watts>167</Watts></TPX></Extensions></Trackpoint><Trackpoint><Time>2008-03-03T13:59:44Z</Time><Position><LatitudeDegrees>35.867902</LatitudeDegrees><LongitudeDegrees>-78.914791</LongitudeDegrees></Position><AltitudeMeters>81.849</AltitudeMeters><DistanceMeters>6259.835</DistanceMeters><Cadence>66</Cadence><Extensions><TPX xmlns=\"http://www.garmin.com/xmlschemas/ActivityExtension/v2\"><Watts>161</Watts></TPX></Extensions></Trackpoint><Trackpoint><Time>2008-03-03T13:59:45Z</Time><Position><LatitudeDegrees>35.867841</LatitudeDegrees><LongitudeDegrees>-78.914793</LongitudeDegrees></Position><AltitudeMeters>81.849</AltitudeMeters><DistanceMeters>6266.723</DistanceMeters><Cadence>66</Cadence><Extensions><TPX xmlns=\"http://www.garmin.com/xmlschemas/ActivityExtension/v2\"><Watts>169</Watts></TPX></Extensions></Trackpoint><Trackpoint><Time>2008-03-03T13:59:46Z</Time><Position><LatitudeDegrees>35.867776</LatitudeDegrees><LongitudeDegrees>-78.914793</LongitudeDegrees></Position><AltitudeMeters>82.330</AltitudeMeters><DistanceMeters>6273.886</DistanceMeters><Cadence>66</Cadence><Extensions><TPX xmlns=\"http://www.garmin.com/xmlschemas/ActivityExtension/v2\"><Watts>170</Watts></TPX></Extensions></Trackpoint><Trackpoint><Time>2008-03-03T13:59:47Z</Time><Position><LatitudeDegrees>35.867712
